vi "tearDown.vi"(8 "error in (no error)":errorcluster, 11 "reference in":refnum<class "testcase-Broadcast Registry.lvclass">) -> (0 "error out":errorcluster, 3 "reference out":refnum<class "testcase-Broadcast Registry.lvclass">)   [LabVIEW 2017, in "testcase-Broadcast Registry.lvclass"]
doc: "tearDown runs after the test method has completed. Use this method to clean up any operations or references that were opened by setUp or the test method. Unit tests should be independent of other unit tests so this VI should ensure that the next test can run in a 'clean' test environment."
uses:
  testcase-Broadcast Registry.lvclass
  testcase-Broadcast Registry.lvclass/testcase-Broadcast Registry.ctl
  src/user.lib/_NEVSTOP/Communicable State Machine(CSM)/Communicable State Machine.lvlib
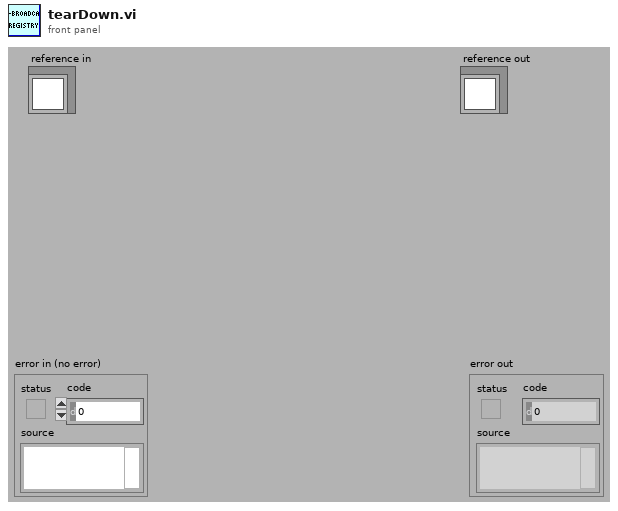
[diagram p1: front panel]
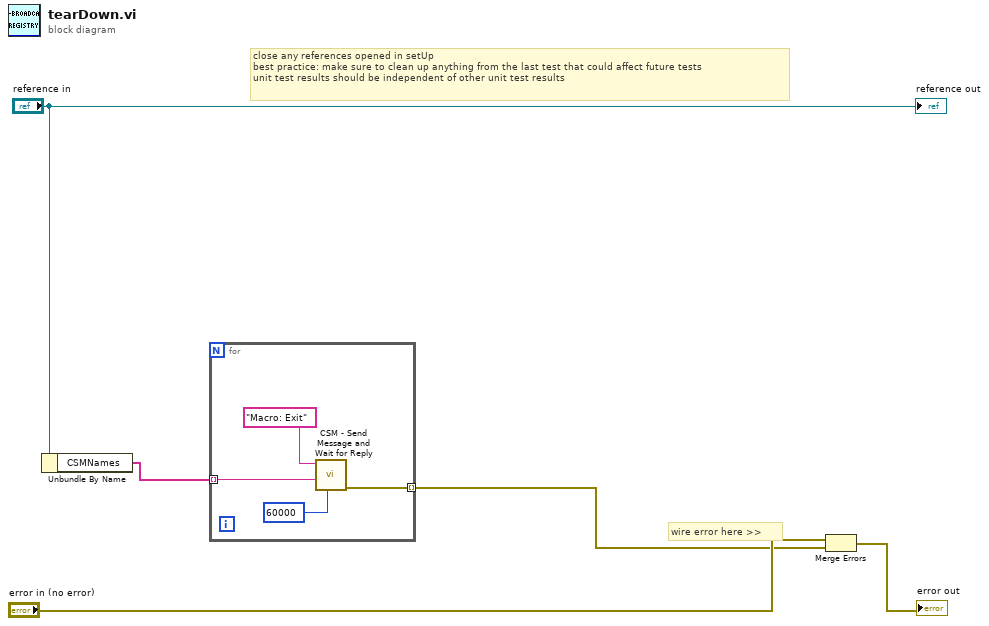
[diagram p0: block diagram]
diagram:
  # "wire error here >>"
  # "close any references opened in setUp\nbest practice: make sure to clean up anything from the last test that could affect future tests\nunit test results should be independent of other unit test results"
  n1 = Unbundle By Name("reference in") -> ("CSMNames"=w2:string[])
  n2 = for {
    tunnel: w2 -> [w8] mode=indexing
    tunnel: [w7] -> w1 mode=indexing
    n3 = call "CSM - Send Message and Wait for Reply.vi"("Response Timeout (-2 Using Global Settings)"=60000, "Target Module"=w8, "State"="Macro: Exit") -> ("error out"=w7:errorcluster)  [unwired: 6 in, 2 out]
  }
  n4 = Merge Errors("error in (no error)", w1) -> (→"error out":errorcluster)
  "reference out" <- "reference in"
